vi "EncoderPID.vi"(4 "Reset":bool, 7 "PID gains":T5={"proportional gain (Kc)"=1.0, "integral time (Ti, min)"=0.01, "derivative time (Td, min)"=0.0} {"derivative time (Td, min)" format="%.3f"; "integral time (Ti, min)" format="%.3f"; "proportional gain (Kc)" format="%.3f"}, 8 "Wheel":dbl, 9 "EncoderRef":T1={"DevStatus"={"status"=FALSE, "code"=0, "source"=""}, "EncoderIndex"=enum."Invalid", "CounterIndex"=enum."Ctr 1", "DistancePerCount"=2.0, "Decoding Type"=enum."4x"}) -> (0 "Encoder Measured Speed":dbl, 1 "Speed Target":dbl, 2 "dt":dbl, 3 "output":dbl format="%.2f")   [LabVIEW 2013]
uses:
  <vilib>/Rock Robotics/WPI/Encoder/WPI_EncoderDevRef.ctl
  <vilib>/Rock Robotics/SystemInterfaces/Encoder/FPGA_EncoderIdx.ctl
  <vilib>/Rock Robotics/SystemInterfaces/Counter/FPGA_CounterCtrSystemIndex.ctl
  <vilib>/Rock Robotics/WPI/Encoder/WPI_EncoderType.ctl
panel:
  in  "Threshold":dbl
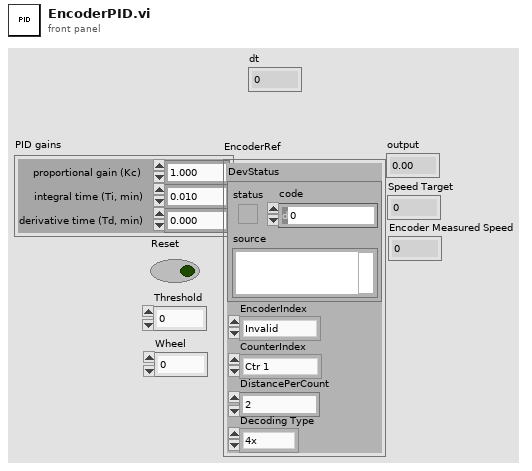
[diagram p1: front panel]
types:
  T1 = typedef "WPI_EncoderDevRef.ctl" = cluster{"DevStatus":errorcluster, "EncoderIndex":T2, "CounterIndex":T3, "DistancePerCount":dbl, "Decoding Type":T4}
  T2 = typedef "FPGA_EncoderIdx.ctl" = enum8{"Enc 0", "Enc 1", "Enc 2", "Enc 3", "Invalid"}
  T3 = typedef "FPGA_CounterCtrSystemIndex.ctl" = enum8{"Ctr 0", "Ctr 1", "Ctr 2", "Ctr 3", "Ctr 4", "Ctr 5", "Ctr 6", "Ctr 7", "Invalid"}
  T4 = typedef "WPI_EncoderType.ctl" = enum16{"1x", "2x", "4x"}
  T5 = cluster{"proportional gain (Kc)":dbl, "integral time (Ti, min)":dbl, "derivative time (Td, min)":dbl}
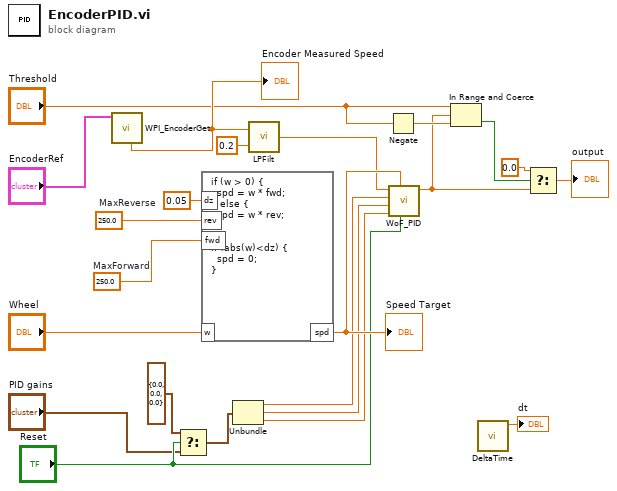
[diagram p0: block diagram]
diagram:
  w19 = 250.0  # MaxReverse
  w20 = 250.0  # MaxForward
  n1 = call <vilib>:"WPI_EncoderGet.vi"("EncoderDevRef"="EncoderRef") -> ("Rate"=w14:dbl)  [unwired: 5 in, 5 out]
  "Encoder Measured Speed" <- w14
  n2 = Select(t=T5 {"proportional gain (Kc)"=0.0, "integral time (Ti, min)"=0.0, "derivative time (Td, min)"=0.0}, s="Reset", f="PID gains") -> (s? t:f=w3:T5)
  n3 = formula code="if (w > 0) {\n  spd = w * fwd;\n} else {\n  spd = w * rev;\n}\n\nif (abs(w)<dz) {\n  spd = 0;\n}"("rev"=w19, "fwd"=w20, "w"="Wheel", "dz"=0.05 ("input variable")) -> ("spd"=w18:dbl)
  "Speed Target" <- w18
  n4 = Unbundle(w3) -> ("proportional gain (Kc)"=w17:dbl, "integral time (Ti, min)"=w16:dbl, "derivative time (Td, min)"=w15:dbl)
  n5 = call "LPFilt.vi"("LP%"=0.2, "Input"=w14) -> ("Filtered"=w13:dbl)
  n6 = Negate(x="Threshold") -> (-x=w11:dbl)
  n7 = call "WoF_PID.vi"("Reset"="Reset", "Desired"=w18, "D"=w15, "I"=w16, "P"=w17, "Actual"=w13) -> ("Control Effort"=w8:dbl)  [unwired: 5 in]
  n8 = In Range and Coerce(upper limit="Threshold", x=w8, lower limit=w11) -> (In Range?=w9:bool)  [unwired: 1 out]
  n9 = call "DeltaTime.vi"() -> ("dt"=→"dt":dbl)  [unwired: 11 in]
  n10 = Select(t=0.0, s=w9, f=w8) -> (s? t:f=→"output":dbl)
